vi "UHR-Fleezers Control (host) - 10.6.vi"() -> ()   [LabVIEW 2011] (continued)
                                n777 = property on="Green Laser ON/Interlacing" class="Bool (strict)"("Val(Sgnl)"=TRUE ("Green Laser ON/Interlacing")) -> ()  [unwired: 2 in, 2 out]
                                }
                                }
                                }
                                frame #2 {
                                n778 = Wait (ms)(milliseconds to wait=u32 500) -> ()  [unwired: 1 out]
                                }
                                frame #3 {
                                n779 = local write "Start Saving"("Save at end (5, 6)") -> ()
                                }
                                }
                                }
                                frame #2 {
                                n780 = local read "Bead Sep. Int. Time (s)"() -> (w1214:dbl)
                                n781 = Multiply(x=w1214, y=1000.0) -> (x*y=w1213:dbl)
                                n782 = Wait (ms)(milliseconds to wait=w1213) -> ()  [unwired: 1 out]
                                }
                                frame #3 {
                                n783 = property on="Remove Offset" class="Bool (strict)"("Val(Sgnl)"=TRUE ("Value (Signaling)")) -> ()  [unwired: 2 in, 2 out]
                                }
                                }
                                }
                                }
                                }
                                }
                                }
                                }
                                }
                                frame "2", Default {
                                }
                              }
                            }
                          }
                        }
                      }
                      "Tether" <- "Tether Alarm?"
                    }
                  }
                }
                frame #2 {
                  n784 = local read "Oscillate Set 1"() -> (w1221:bool)
                  n785 = local read "Stop All"() -> (w1219:bool)
                  n786 = Or(x=w1221, y=w1216) -> (x .or. y?=w1218:bool)
                  n787 = Not(x=w1218) -> (.not. x?=w1220:bool)
                  n788 = Compound Arithmetic op=OR(w1219, w1220) -> (w1217:bool)
                }
              }
              n789 = node-c288() -> ()  [unwired: 2 out]
            }
            n790 = node-c288(w1062) -> ()  [unwired: 1 out]
          }
        }
      }
      event "Fl. Triggered...": Value Change {
        n791 = event-data() -> ()  [unwired: 7 out]
        n792 = case shown="True" "Fl. Triggered..." {
          frame False {
          }
          frame True {
            n793 = node-c288() -> (w1231:T21)  [unwired: 4 out]
            n794 = timed-loop {
              timing: w1231 -> [_]
              timing-out: [_] -> w1230
              tunnel: "Action" -> [w1235]
              shift-right: [w1232] -> _
              shift-left: u8 255 -> [w1234]
              stop <- w1236 stop-if-true
              n795 = node-c288() -> ()  [unwired: 2 out]
              n796 = flat-sequence {
                tunnel: w1235 -> [w1248]
                tunnel: w1234 -> [w1245]
                tunnel: [w1244] -> w1233
                tunnel: [w1334] -> w1236
                tunnel: w1233 -> [w1333]
                tunnel: [w1333] -> w1232
                frame #0 {
                  n797 = local read "Delta Fl. 2"() -> (w1239:dbl)
                  n798 = local read "Delta Fl. 1"() -> (w1240:dbl)
                  n799 = Select(t=w1240, s="APD to Watch", f=w1239) -> (s? t:f=w1238:dbl)
                  n800 = Multiply(x="Fl. Delta Thresh. (kHz)", y=1000.0) -> (x*y=w1247:dbl)
                  n801 = Greater?(x=w1238, y=w1247) -> (0:w1242:bool)
                  n802 = Or(x="Force Yank", y=w1242) -> (x .or. y?=w1243:bool)
                  n803 = case shown="True" w1243 {
                    tunnel: w1248 -> [_ w1258]
                    tunnel: w1245 -> [w1250 w1254]
                    tunnel: [w1250 w1251] -> w1244
                    frame False {
                    }
                    frame True {
                      n804 = flat-sequence {
                        tunnel: w1255 -> [w1264]
                        tunnel: [w1264] -> w1259
                        tunnel: w1258 -> [w1263]
                        tunnel: [w1263] -> w1257
                        tunnel: [w1262] -> w1256
                        tunnel: w1254 -> [w1261]
                        tunnel: [w1260] -> w1253
                        tunnel: w1259 -> [w1289]
                        tunnel: w1257 -> [w1288]
                        tunnel: w1256 -> [w1287]
                        tunnel: w1253 -> [w1286]
                        tunnel: [w1286] -> w1252
                        tunnel: w1252 -> [w1331]
                        tunnel: [w1331] -> w1251
                        frame #0 {
                          n805 = call <vilib>:"Beep.vi"() -> ()  [unwired: 3 in, 9 out]
                          n806 = local write "Waiting"(FALSE ("Waiting")) -> ()
                          n807 = Increment(x=w1261) -> (x+1=w1260:u8)
                          n808 = case shown="\"Yank\"" w1263 {
                            tunnel: w1260 -> [_ _ w1270]
                            frame "Image" {
                              n809 = property on="Confocal Image" class="Bool (strict)"("Val(Sgnl)"=TRUE ("Value (Signaling)")) -> ()  [unwired: 2 in, 2 out]
                            }
                            frame "Alarm", Default {
                            }
                            frame "Yank" {
                              n810 = flat-sequence {
                                tunnel: w1270 -> [w1273]
                                tunnel: [w1272] -> w1269
                                tunnel: ["N Array El"] -> w1268
                                tunnel: w1269 -> [w1283]
                                tunnel: w1268 -> [w1279]
                                frame #0 {
                                n811 = Multiply(x="Yank Delay (s)", y=1000.0) -> (x*y=w1276:dbl)
                                n812 = Quotient & Remainder(x=w1273, y="N Array El") -> (x-y*floor(x/y)=w1272:u8)  [unwired: 1 out]
                                n813 = Wait (ms)(milliseconds to wait=w1276) -> ()  [unwired: 1 out]
                                }
                                frame #1 {
                                n814 = Random Number (0-1)() -> (number: 0 to 1=w1280:dbl)
                                n815 = Multiply(x=w1279, y=w1280) -> (x*y=w1278:dbl)
                                n816 = Round Toward -Infinity(1:w1278) -> (0:w1277:dbl)
                                n817 = Select(t=w1277, s="Random Choice", f=w1283) -> (s? t:f=w1281:dbl)
                                n818 = Index Array(array="Yank to Delta Array (MHz)", index=w1281) -> (element=w1284:dbl)
                                n819 = property on="Trap Delta (MHz)" class="DigNum (strict)"("Val(Sgnl)"=w1284) -> ()  [unwired: 2 in, 2 out]
                                }
                              }
                            }
                          }
                          n820 = local read "Time (s)"() -> (w1262:dbl)
                          "Fl. High" <- TRUE ("Yanking")
                        }
                        frame #1 {
                          n821 = node-c288() -> (w1291:T21)  [unwired: 4 out]
                          n822 = timed-loop {
                            timing: w1291 -> [_]
                            timing-out: [_] -> w1290
                            tunnel: w1289 -> [w1307]
                            tunnel: w1288 -> [w1305]
                            tunnel: w1287 -> [w1304]
                            stop <- w1306 stop-if-true
                            n823 = node-c288() -> ()  [unwired: 2 out]
                            n824 = local read "Fl. Delta Thresh. (kHz)"() -> (w1299:dbl)
                            n825 = local read "Fl. Triggered..."() -> (w1308:bool)
                            n826 = local read "Delta Fl. 1"() -> (w1295:dbl)
                            n827 = local read "Delta Fl. 2"() -> (w1293:dbl)
                            n828 = local read "Stop All"() -> (w1302:bool)
                            n829 = local read "APD to Watch"() -> (w1294:bool)
                            n830 = Select(t=w1295, s=w1294, f=w1293) -> (s? t:f=w1292:dbl)
                            n831 = Not(x=w1308) -> (.not. x?=w1303:bool)
                            n832 = Multiply(x=w1299, y=1000.0) -> (x*y=w1298:dbl)
                            n833 = Negate(x=w1298) -> (-x=w1297:dbl)
                            n834 = Less?(x=w1292, y=w1297) -> (x < y?=w1301:bool)
                            n835 = Compound Arithmetic op=OR(w1301, w1302, w1303, "Force Reset") -> (w1306:bool)
                            n836 = case shown="True" w1306 {
                              tunnel: w1307 -> [_ w1319]
                              tunnel: w1305 -> [_ w1318]
                              tunnel: w1304 -> [_ w1316]
                              frame False {
                              }
                              frame True {
                                n837 = case shown="\"Yank\"" w1318 {
                                tunnel: w1319 -> [_ w1320]
                                frame "Image", Default {
                                }
                                frame "Yank" {
                                n838 = flat-sequence {
                                tunnel: [w1325] -> w1321
                                tunnel: w1320 -> [w1325]
                                tunnel: w1321 -> [w1326]
                                frame #0 {
                                n839 = local read "Yank Delay (s)"() -> (w1324:dbl)
                                n840 = Multiply(x=w1324, y=1000.0) -> (x*y=w1322:dbl)
                                n841 = Wait (ms)(milliseconds to wait=w1322) -> ()  [unwired: 1 out]
                                }
                                frame #1 {
                                n842 = property on="Trap Delta (MHz)" class="DigNum (strict)"("Val(Sgnl)"=w1326) -> ()  [unwired: 2 in, 2 out]
                                }
                                }
                                }
                                }
                                n843 = local read "Time (s)"() -> (w1317:dbl)
                                n844 = Subtract(x=w1317, y=w1316) -> (x-y=w1313:dbl)
                                "Duration (s)" <- w1313
                                n845 = Number To Decimal String(number=w1313, width (-)=i16 0) -> (decimal integer string=w1311:string)
                                n846 = Concatenate Strings(w1311, " s fluorescence event." ("string")) -> (w1309:string)
                                n847 = local read "Messages"() -> (w1315:string)
                                n848 = call "Update messages.vi"("Message to add"=w1309, "Old message string"=w1315) -> ("New message string"=w1314:string)
                                n849 = call <vilib>:"Beep.vi"() -> ()  [unwired: 3 in, 9 out]
                                n850 = local write "Messages"(w1314) -> ()
                              }
                            }
                            n851 = node-c288() -> ()  [unwired: 2 out]
                          }
                          n852 = node-c288(w1290) -> ()  [unwired: 1 out]
                        }
                        frame #2 {
                          n853 = local write "Fl. High"(FALSE ("Yanking")) -> ()
                        }
                      }
                      n854 = local read "Trap Delta (MHz)"() -> (w1255:dbl)
                    }
                  }
                }
                frame #1 {
                  n855 = local read "Stop All"() -> (w1337:bool)
                  n856 = local read "Fl. Triggered..."() -> (w1335:bool)
                  n857 = Not(x=w1335) -> (.not. x?=w1336:bool)
                  n858 = Or(x=w1336, y=w1337) -> (x .or. y?=w1334:bool)
                  n859 = Not(x=w1334) -> (.not. x?=→"Waiting":bool)
                }
              }
              n860 = node-c288() -> ()  [unwired: 2 out]
            }
            n861 = node-c288(w1230) -> ()  [unwired: 1 out]
          }
        }
      }
      event "Stop All": Value Change {
        n862 = event-data() -> ()  [unwired: 7 out]
        n863 = local read "Stop All"() -> (w1343:bool)
      }
    }
    n864 = node-c288() -> ()  [unwired: 2 out]
  }
  n865 = timed-loop "Control parameters (event loop)" {
    tunnel: w50 -> [w1352]
    shift-right: [w1351] -> _
    shift-left: errorcluster {"status"=FALSE, "code"=0, "source"=""} ("error out") -> [w1350]
    tunnel: [w1349] -> _
    timing: w92 -> [_]
    timing-out: [_] -> w91
    tunnel: w64 -> [w1348]
    tunnel: w4 -> [w1347]
    tunnel: w3 -> [w1346]
    tunnel: w2 -> [w1345]
    tunnel: w1 -> [w1344]
    stop <- w1349 stop-if-true
    n866 = node-c288() -> ()  [unwired: 2 out]
    n867 = event shown="[56] \"Retract Pump 3\": Value Change" {
      selector: _ -> [_ _ _ _ _ _ _ _ _ _ _ _ _ _ _ _ _ _ _ _ _ _ _ _ _ _ _ _ _ _ _ _ _ _ _ _ _ _ _ _ _ _ _ _ _ _ _ _ _ _ _ _ _ _ _ _ _ _ _ _ _ _ _ _ _ _ _ _ _ _ _ _ _]
      dyn-events: _ -> [_ _ _ _ _ _ _ _ _ _ _ _ _ _ _ _ _ _ _ _ _ _ _ _ _ _ _ _ _ _ _ _ _ _ _ _ _ _ _ _ _ _ _ _ _ _ _ _ _ _ _ _ _ _ _ _ _ _ _ _ _ _ _ _ _ _ _ _ _ _ _ _ _]
      timeout: _ -> [_ _ _ _ _ _ _ _ _ _ _ _ _ _ _ _ _ _ _ _ _ _ _ _ _ _ _ _ _ _ _ _ _ _ _ _ _ _ _ _ _ _ _ _ _ _ _ _ _ _ _ _ _ _ _ _ _ _ _ _ _ _ _ _ _ _ _ _ _ _ _ _ _]
      tunnel: w1352 -> [w1390 _ _ _ w1428 _ w1450 _ _ _ _ w1516 _ _ w1559 w1565 w1570 w1576 w1612 w1630 w1637 w1648 w1652 w1663 w1674 w1685 w1696 w1707 w1718 w1745 w1839 w1846 w1884 _ w1919 w1923 w1934 w1938 w1942 _ w1950 _ _ _ _ _ _ _ _ _ _ _ _ _ _ _ _ _ w2328 _ w2345 _ w2352 w2370 _ w2377 w2385 w2400 w2411 w2414 w2419 _ w2438]
      tunnel: [w1389 _ _ _ w1418 _ w1449 _ _ w1481 _ w1495 _ _ w1558 w1561 w1567 w1573 w1611 w1628 w1636 w1646 _ w1657 w1668 w1679 w1690 w1701 w1712 w1743 w1837 w1844 w1882 _ w1917 w1921 w1924 w1936 w1940 _ w1948 _ _ _ _ _ _ _ _ _ _ _ _ _ _ _ _ _ w2326 _ _ _ _ w2367 _ _ _ _ _ _ _ _ _] -> w1351
      tunnel: w1350 -> [w1388 _ _ _ w1427 _ w1448 _ _ w1481 _ w1515 _ _ w1557 w1560 w1566 w1572 w1610 w1629 w1635 w1647 w1651 w1662 w1673 w1684 w1695 w1706 w1717 w1744 w1838 w1845 w1883 _ w1918 w1922 w1933 w1937 w1941 _ w1949 _ _ _ _ _ _ _ _ _ _ _ _ _ _ _ _ _ w2327 _ w2344 _ w2351 w2369 _ w2376 w2384 w2399 w2410 w2413 w2418 _ w2437]
      tunnel: [_ _ _ _ _ _ _ _ _ w1480 _ _ _ _ _ _ _ _ _ _ _ _ _ _ _ _ _ _ _ _ _ _ _ _ _ _ _ _ _ _ _ _ _ _ _ _ _ _ _ _ _ _ _ _ _ _ _ _ _ _ _ _ _ _ _ _ _ _ _ _ _ _ _] -> w1349
      tunnel: [_ _ _ _ _ _ _ "Round T1 X" _ _ _ _ _ _ _ _ _ _ _ _ _ _ _ _ _ _ _ _ _ _ _ _ _ _ _ _ _ _ _ _ _ _ _ _ _ _ _ _ _ _ _ _ _ _ _ _ _ _ _ _ _ _ _ _ _ _ _ _ _ _ _ _ _] -> _
      tunnel: [_ _ _ "Adjust Scale\nto Mean" _ _ _ _ _ _ _ _ _ _ _ _ _ _ _ _ _ "Test ttrig" _ _ _ _ _ _ _ _ _ _ _ _ _ _ _ _ _ _ _ _ _ _ _ _ _ _ "Flush Sample" "Flush Pump 3" "Flush Pump 1" "Clear Volume" _ _ _ _ _ _ _ _ _ _ _ _ _ _ _ _ _ _ _ _ _] -> _
      tunnel: [_ _ _ _ _ _ _ _ "Round T2 X" _ "Delayed Interlace Start" _ _ _ _ _ _ _ _ _ _ _ _ _ _ _ _ _ _ _ _ _ _ _ _ _ _ _ _ _ _ _ _ _ _ _ _ _ _ _ _ _ _ _ _ _ _ _ _ _ _ _ _ _ _ _ _ _ _ _ _ _ _] -> _
      tunnel: w1348 -> [_ _ _ _ _ _ _ _ _ _ _ _ _ _ _ _ _ _ _ _ _ _ _ _ _ _ _ _ _ _ _ _ _ _ _ _ _ _ _ _ _ _ _ _ w2107 w2114 w2121 w2126 w2135 _ _ w2241 _ _ _ _ _ _ _ _ _ _ _ _ _ _ _ _ _ _ _ _ _]
      tunnel: w1347 -> [_ _ _ _ _ _ _ _ _ _ _ _ _ _ _ _ _ _ _ _ _ _ _ _ _ _ _ _ _ _ _ _ _ _ _ _ _ _ _ _ _ _ w2024 _ _ _ _ _ _ w2179 _ _ w2247 _ w2256 _ w2270 _ _ _ _ _ _ _ _ _ _ _ _ _ _ _ _]
      tunnel: w1346 -> [_ _ _ _ _ _ _ _ _ _ _ _ _ _ _ _ _ _ _ _ _ _ _ _ _ _ _ _ _ _ _ _ _ _ _ _ _ _ _ _ _ _ _ _ _ _ _ _ _ _ _ _ _ _ _ _ _ _ _ _ _ _ _ _ _ _ _ _ _ _ _ _ _]
      tunnel: w1345 -> [_ _ _ _ _ _ _ _ _ _ _ _ _ _ _ _ _ _ _ _ _ _ _ _ _ _ _ _ _ _ _ _ _ _ _ _ _ _ _ _ _ w1961 _ _ _ _ _ _ _ _ w2209 _ _ w2252 _ w2263 _ w2295 _ _ _ _ _ _ _ _ _ _ _ _ _ _ _]
      tunnel: w1344 -> [_ _ _ _ _ _ _ _ _ _ _ _ _ _ _ _ _ _ _ _ _ _ _ _ _ _ _ _ _ _ _ _ _ _ _ _ _ _ _ _ _ _ _ _ _ _ _ _ _ _ _ _ _ _ _ _ _ _ _ _ _ _ _ _ _ _ _ _ _ _ _ _ _]
      event "AI Count (ticks)", "Sets to FIFO (Traps)", "Save ave N", "FPGA Ave.", "# Samples/channel", "N sets to save": Value Change {
        # "So that if 'Save ave N' is updated, the AOD scanning code updates too."
        n868 = event-data() -> ()  [unwired: 6 out]
        n869 = local read "AI Count (ticks)"() -> (w1370:u32)
        n870 = Boolean To (0,1)(Boolean="Sets to FIFO (Traps)") -> (0, 1=w1380:cluster{"Set 1":i16, "Set 2":i16, "Set 3":i16})
        n871 = xnode "Read/Write Control"("FPGA VI Reference In"=w1390, "error in"=w1388, "ai count"=w1370, "AI1 Sets to FIFO"="Sets to FIFO (Traps)", "N of AI1 Int Acq Sets"="N Acq Sets (Traps + Fl.)") -> ("error out"=w1389:errorcluster)  [unwired: 1 out]
        n872 = Cluster To Array(cluster=w1380) -> (array=w1379:i16[])
        n873 = To Unsigned Long Integer(number=w1379) -> (unsigned 32bit integer=w1359:u32[])
        n874 = local read "Scan steps (AOD)"() -> (w1381:u64)
        n875 = Multiply(x=w1370, y="N Acq Sets (Traps + Fl.)") -> (x*y=w1368:u32)
        n876 = Divide(x=40000000.0, y=w1370) -> (x/y=w1362:dbl)
        "AI rate (Hz)" <- w1362
        "Ave. Rate (Hz)" <- w1362
        n877 = Add Array Elements(numeric array=w1359) -> (sum=w1371:u32)
        "Trap Sets" <- w1371
        n878 = Reciprocal(x=w1362) -> (1/x=→"Ave. Period (s)":dbl)
        n879 = property on="Scan steps (AOD)" class="DigNum (strict)"("Val(Sgnl)"=w1381) -> ()  [unwired: 2 in, 2 out]
        n880 = Divide(x=w1362, y="N Acq Sets (Traps + Fl.)") -> (x/y=w1385:dbl)
        "Data Rate (Hz)" <- w1385
        n881 = Reciprocal(x=w1385) -> (1/x=→"Data Period (s)":dbl)
        n882 = local read "Save ave N"() -> (w1384:dbl)
        n883 = Divide(x=w1385, y=w1384) -> (x/y=w1383:dbl)
        "Save Data Rate (Hz)" <- w1383
        n884 = Reciprocal(x=w1383) -> (1/x=→"Save Data Period (s)":dbl)
        n885 = Multiply(x=w1368, y="# Samples/trap") -> (x*y=w1366:u32)
        "Counts/DMA" <- w1366
        n886 = property on="Trap Disp. Downsample" class="DigNum (strict)"("Maximum"="# Samples/trap") -> ()  [unwired: 2 in, 2 out]
        n887 = Multiply(x=w1371, y="# Samples/trap") -> (x*y=w1360:u32)
        "# Samples/channel" <- w1360
        n888 = Multiply(x=w1360, y=u32 8) -> (x*y=→"Trap AI Elements/DMA read":u32)
        n889 = local read "APD Int. Count"() -> (w1367:u32)
        n890 = Multiply(x=w1360, y=u32 3) -> (x*y=→"Trap Pos Elements/DMA read":u32)
        n891 = Divide(x=w1366, y=w1367) -> (x/y=w1357:dbl)
        "APD Samples/FIFO Acq." <- w1357
        n892 = Divide(x=w1366, y=40000000.0) -> (x/y=w1364:dbl)
        "DMA Update Period (s)" <- w1364
        n893 = Multiply(x=2.0, y=w1357) -> (x*y=→"APD Elements/DMA read":dbl)
        n894 = property on="APD Disp. Downsample" class="DigNum (strict)"("Maximum"=w1357) -> ()  [unwired: 2 in, 2 out]
        n895 = local read "N sets to save"() -> (w1377:u32)
        n896 = Multiply(x=w1364, y=w1377) -> (x*y=→"Total Time (s)":dbl)
        "FPGA Averaging" <- FALSE ("FPGA Averaging")
      }
      event "Remove Offset": Value Change {
        n897 = event-data() -> ()  [unwired: 7 out]
        n898 = local write "Remove Offset"(FALSE ("Remove Offset")) -> ()
        n899 = local read "Bead Mean (nm)"() -> (w1392:dbl)
        n900 = local read "Offset (nm)"() -> (w1393:dbl)
        n901 = Add(x=w1392, y=w1393) -> (x+y=w1391:dbl)
        n902 = local write "Offset (nm)"(w1391) -> ()
        n903 = disable-structure shown="Disabled" {
          frame Disabled {
            n904 = local read "Bead Mean (nm)"() -> (w1398:dbl)
            n905 = Add(y=w1398) -> (x=w1397:dbl, x+y=w1396:dbl)
            n906 = Subtract(x=w1398, y=w1397) -> (x-y=w1395:dbl)
            n907 = property on="Bead Separation" class="WFChart (strict)"("YScale.Minimum"=w1395) -> ()  [unwired: 2 in, 2 out]
            n908 = property on="Bead Separation" class="WFChart (strict)"("YScale.Maximum"=w1396) -> ()  [unwired: 2 in, 2 out]
          }
          frame Enabled {
          }
        }
      }
      event "Detector Type": Value Change {
        n909 = event-data() -> ()  [unwired: 7 out]
        n910 = local read "AI labels"() -> (w1399:string[])
        n911 = property on="High Res. Display" class="Ring (strict)"("Strings []"=w1399) -> ()  [unwired: 2 in, 2 out]
        n912 = Build Array (concatenate)(w1399, "none") -> (w1400:string[])
        n913 = property on="FFT 1 Choice 1" class="Ring (strict)"("Strings []"=w1400) -> ()  [unwired: 2 in, 2 out]
        n914 = property on="FFT 1 Choice 2" class="Ring (strict)"("Strings []"=w1400) -> ()  [unwired: 2 in, 2 out]
        n915 = property on="FFT 2 Choice 1" class="Ring (strict)"("Strings []"=w1400) -> ()  [unwired: 2 in, 2 out]
        n916 = property on="FFT 2 Choice 2" class="Ring (strict)"("Strings []"=w1400) -> ()  [unwired: 2 in, 2 out]
        n917 = Bundle("APD 1", "APD 2") -> (w1403:cluster{string, string})  [unwired: 1 out]
        n918 = Cluster To Array(cluster=w1403) -> (array=w1401:string[])
        n919 = Build Array (concatenate)(w1401, w1400) -> (w1405:string[])
        n920 = Array Size(array=w1405) -> (size(s)=w1406:i32)
        n921 = property on="Signals to Plot" class="LstBox (strict)"("Item Names"=w1405) -> ()  [unwired: 2 in, 2 out]
        n922 = property on="Signals to Plot" class="LstBox (strict)"("Number of Rows"=w1406) -> ()  [unwired: 2 in, 2 out]
        n923 = property on="All Signals" class="WFChart (strict)"("LegNumRows"=w1406) -> ()  [unwired: 2 in, 2 out]
      }
      event "Adjust Scale\nto Mean": Value Change {
        n924 = event-data() -> ()  [unwired: 7 out]
        n925 = local read "APD 1 Rate (Hz)"() -> (w1415:dbl)
        n926 = Multiply(x=1000.0, y="Above (kHz)") -> (x*y=w1413:dbl)
        n927 = Multiply(x=1000.0, y="Below (kHz)") -> (x*y=w1411:dbl)
        n928 = Add(x=w1413, y=w1415) -> (x+y=w1408:dbl)
        n929 = Subtract(x=w1415, y=w1411) -> (x-y=w1409:dbl)
        n930 = property on="APD Chart" class="WFChart (strict)"("YScale.Minimum"=w1409) -> ()  [unwired: 2 in, 2 out]
        n931 = property on="APD Chart" class="WFChart (strict)"("YScale.Maximum"=w1408) -> ()  [unwired: 2 in, 2 out]
      }
      event "Phase adj. (AI1)", "+ phase (AI1)", "- phase (AI1)": Value Change {
        n932 = event-data() -> ()  [unwired: 7 out]
        n933 = Negate(x="Phase adj. (AI1)") -> (-x=w1425:i16)
        n934 = Select(t=w1425, s="- phase (AI1)", f="Phase adj. (AI1)") -> (s? t:f=w1424:i16)
        n935 = xnode "Read/Write Control"("FPGA VI Reference In"=w1428, "error in"=w1427, "Phase count adjustment"=w1424) -> ("FPGA VI Reference Out"=w1423:T19, "error out"=w1422:errorcluster)
        n936 = Or(x="- phase (AI1)", y="+ phase (AI1)") -> (x .or. y?=w1419:bool)
        n937 = xnode "Read/Write Control"("FPGA VI Reference In"=w1423, "error in"=w1422, "+ phase"=w1419) -> ("error out"=w1418:errorcluster)  [unwired: 1 out]
      }
      event "Signals to Plot": Double Click {
        w1431 = u32 9868950 ("Color Box")
        n938 = event-data() -> ("Row"=w1433:i32)  [unwired: 9 out]
        n939 = property on="All Signals" class="WFChart (strict)"("Active Plot"=w1433) -> (error out=w1444:errorcluster)  [unwired: 2 in, 1 out]
        n940 = property on="All Signals" class="WFChart (strict)" props=["Plot", "Visible?", "Plot", "Plot Color"](error in=w1444) -> (error out=w1443:errorcluster, "Plot.Visible?"=w1442:bool)  [unwired: 1 in, 2 out]
        n941 = Select(t=FALSE ("Plot.Visible"), s=w1442, f=TRUE ("Plot.Visible")) -> (s? t:f=w1437:bool)
        n942 = property on="All Signals" class="WFChart (strict)"(error in=w1443, "Plot.Visible?"=w1437) -> (error out=w1439:errorcluster)  [unwired: 1 in, 1 out]
        n943 = property on="All Signals" class="WFChart (strict)"(error in=w1439) -> (error out=w1434:errorcluster, "Plot.Plot Color"=w1438:u32)  [unwired: 1 in, 1 out]
        n944 = property on="Signals to Plot" class="LstBox (strict)"(error in=w1434, "Active Row"=w1433) -> (error out=w1432:errorcluster)  [unwired: 1 in, 1 out]
        n945 = Select(t=w1438, s=w1437, f=u32 0) -> (s? t:f=w1435:u32)
        n946 = property on="Signals to Plot" class="LstBox (strict)"(error in=w1432, "CellFontColor"=w1435, "SelColor"=w1431, "CellBG"=w1431, "CellFontSize"=u32 20 ("Active Row:Cell Font:Size"), "CellFontBold"=TRUE ("Active Row:Cell Font:Bold")) -> ()  [unwired: 1 in, 2 out]
      }
      event "BD 1 Frequency 1 (MHz)", "BD 1 Frequency 2 (MHz)", "BD 1 Frequency 3 (MHz)", "BD 2 Frequency 1 (MHz)", "BD 2 Frequency 2 (MHz)", "BD 2 Frequency 3 (MHz)", "Trap Delta (MHz)": Value Change {
        n947 = event-data() -> ("CtlRef"=w1447:refnum<vi>)  [unwired: 6 out]
        n948 = control-ref of="Trap Delta (MHz)"() -> (w1446:refnum<vi>)
        n949 = Equal?(x=w1446, y=w1447) -> (x = y?=w1445:bool)
        n950 = case shown="False" "Oscillate Set 1" {
          tunnel: w1450 -> [w1470 _]
          tunnel: [w1469 w1473] -> w1449
          tunnel: w1448 -> [w1468 w1473]
          tunnel: w1445 -> [w1453 _]
          frame False {
            n951 = local read "BD 1 Frequency 2 (MHz)"() -> (w1457:dbl)
            n952 = local read "BD 1 Frequency 1 (MHz)"() -> (w1455:dbl)
            n953 = Subtract(x=w1457, y="Trap Delta (MHz)") -> (x-y=w1454:dbl)
            n954 = Select(t=w1454, s=w1453, f=w1455) -> (s? t:f=w1452:dbl)
            n955 = local read "Y RF Frequency Limits (MHz)"() -> (w1458:T16)
            n956 = local read "X RF Frequency Limits (MHz)"() -> (w1459:T16)
            n957 = local read "BD 1 Frequency 3 (MHz)"() -> (w1471:dbl)
            n958 = local write "BD 1 Frequency 1 (MHz)"(w1452) -> ()
            n959 = local read "BD 2 Frequency 1 (MHz)"() -> (w1462:dbl)
            n960 = local read "BD 2 Frequency 2 (MHz)"() -> (w1461:dbl)
            n961 = local read "BD 2 Frequency 3 (MHz)"() -> (w1472:dbl)
            n962 = call "set RF board frequency - interlace.vi"("Board 2 Frequency Limits"=w1458, "Board 1 Frequency Limits"=w1459, "error in"=w1468, "FPGA VI Reference In"=w1470, "Board 2 Frequency 3 (MHz)"=w1472, "Board 1 Frequency 3 (MHz)"=w1471, "Board 2 Frequency 2 (MHz)"=w1461, "Board 2 Frequency 1 (MHz)"=w1462, "Board 1 Frequency 2 (MHz)"=w1457, "Board 1 Frequency 1  (MHz)"=w1452) -> ("error out"=w1469:errorcluster)  [unwired: 1 out]
            n963 = Subtract(x=w1462, y=w1461) -> (x-y=w1466:dbl)
            n964 = Subtract(x=w1452, y=w1457) -> (x-y=w1467:dbl)
            n965 = Square(x=w1466) -> (x^2=w1464:dbl)
            n966 = Square(x=w1467) -> (x^2=w1465:dbl)
            n967 = Add(x=w1465, y=w1464) -> (x+y=w1463:dbl)
            n968 = Square Root(x=w1463) -> (sqrt(x)=w1460:dbl)
            n969 = local write "Trap Delta (MHz)"(w1460) -> ()
            n970 = property on="Initial delta (MHz)" class="DigNum (strict)"("Val(Sgnl)"=w1460) -> ()  [unwired: 2 in, 2 out]
          }
          frame True {
          }
        }
      }
      event "Round T1 X": Value Change {
        n971 = event-data() -> ()  [unwired: 7 out]
        n972 = local read "BD 1 Frequency 1 (MHz)"() -> (w1476:dbl)
        n973 = Round To Nearest(number=w1476) -> (nearest integer value=w1475:dbl)
        n974 = property on="BD 1 Frequency 1 (MHz)" class="DigNum (strict)"("Val(Sgnl)"=w1475) -> ()  [unwired: 2 in, 2 out]
      }
      event "Round T2 X": Value Change {
        n975 = event-data() -> ()  [unwired: 7 out]
        n976 = local read "BD 1 Frequency 2 (MHz)"() -> (w1478:dbl)
        n977 = Round To Nearest(number=w1478) -> (nearest integer value=w1477:dbl)
        n978 = property on="BD 1 Frequency 2 (MHz)" class="DigNum (strict)"("Val(Sgnl)"=w1477) -> ()  [unwired: 2 in, 2 out]
      }
      event "Stop All": Value Change {
        n979 = event-data() -> ()  [unwired: 7 out]
        n980 = local read "Stop All"() -> (w1480:bool)
      }
      event "Delayed Interlace Start": Value Change {
        n981 = event-data() -> ()  [unwired: 7 out]
        n982 = flat-sequence {
          frame #0 {
            n983 = Multiply(x="Delay to Interlace (s)", y=1000.0) -> (x*y=w1483:dbl)
            n984 = Wait (ms)(milliseconds to wait=w1483) -> ()  [unwired: 1 out]
          }
          frame #1 {
            n985 = property on="Green laser mode" class="RadioBtnsControl (strict)"("Val(Sgnl)"=enum32{"Laser ON", "Laser OFF", "Interlace"}."Interlace" ("Value (Signaling)")) -> ()  [unwired: 2 in, 2 out]
          }
        }
      }
      event "BD 1 Amplitude 1 (%)", "BD 1 Amplitude 2 (%)", "BD 1 Amplitude 3 (%)", "BD 2 Amplitude 1 (%)", "BD 2 Amplitude 2 (%)", "BD 2 Amplitude 3 (%)", "Trap 1 ON", "Trap 2 ON", "Trap 3 ON", "Feedback On/Off", "All FB On/Off": Value Change {
        w1507 = i16 1 ("f")
        n986 = event-data() -> ()  [unwired: 7 out]
        n987 = local write "Trap 1 (ON/OFF)"("Trap 1 ON") -> ()
        n988 = local write "Trap 2 (ON/OFF)"("Trap 2 ON") -> ()
        n989 = Boolean To (0,1)(Boolean="Trap 3 ON") -> (0, 1=w1508:i16)
        n990 = Boolean To (0,1)(Boolean="Trap 1 ON") -> (0, 1=w1509:i16)
        n991 = Boolean To (0,1)(Boolean="Trap 2 ON") -> (0, 1=w1510:i16)
        n992 = Select(t=w1510, s="Trap ON/OFF X or Y Amp?", f=w1507) -> (s? t:f=w1505:i16)
        n993 = Select(t=w1509, s="Trap ON/OFF X or Y Amp?", f=w1507) -> (s? t:f=w1506:i16)
        n994 = Select(t=w1508, s="Trap ON/OFF X or Y Amp?", f=w1507) -> (s? t:f=w1504:i16)
        n995 = Select(t=w1507, s="Trap ON/OFF X or Y Amp?", f=w1510) -> (s? t:f=w1502:i16)
        n996 = Select(t=w1507, s="Trap ON/OFF X or Y Amp?", f=w1509) -> (s? t:f=w1503:i16)
        n997 = Select(t=w1507, s="Trap ON/OFF X or Y Amp?", f=w1508) -> (s? t:f=w1501:i16)
        n998 = And(x="All FB On/Off", y="Feedback On/Off") -> (x .and. y?=w1499:cluster{"Set 1":bool, "Set 2":bool})
        n999 = local read "BD 1 Amplitude 1 (%)"() -> (w1519:dbl)
        n1000 = local read "BD 1 Amplitude 2 (%)"() -> (w1518:dbl)
        n1001 = local read "BD 1 Amplitude 3 (%)"() -> (w1517:dbl)
        n1002 = Unbundle By Name(w1499) -> ("Set 1"=w1494:bool, "Set 2"=w1491:bool)
        n1003 = local read "Y RF Amplitude Limits (%)"() -> (w1487:T16)
        n1004 = local read "X RF Amplitude Limits (%)"() -> (w1488:T16)
        n1005 = local read "BD 2 Amplitude 1 (%)"() -> (w1520:dbl)
        n1006 = local read "BD 2 Amplitude 2 (%)"() -> (w1521:dbl)
        n1007 = local read "BD 2 Amplitude 3 (%)"() -> (w1522:dbl)
        n1008 = And(x="Trap 2 ON", y=w1491) -> (x .and. y?=w1489:bool)
        n1009 = And(x="Trap 1 ON", y=w1494) -> (x .and. y?=w1492:bool)
        n1010 = Multiply(x=w1506, y=w1519) -> (x*y=w1514:dbl)
        n1011 = Multiply(x=w1518, y=w1505) -> (x*y=w1512:dbl)
        n1012 = Multiply(x=w1517, y=w1504) -> (x*y=w1513:dbl)
        n1013 = Multiply(x=w1520, y=w1503) -> (x*y=w1523:dbl)
        n1014 = Multiply(x=w1521, y=w1502) -> (x*y=w1524:dbl)
        n1015 = Multiply(x=w1522, y=w1501) -> (x*y=w1525:dbl)
        n1016 = call "set RF board amplitude - interlace.vi"("Board 2 Amplitude Limits"=w1487, "Board 1 Amplitude Limits"=w1488, "error in"=w1515, "FPGA VI Reference In"=w1516, "Board 2 Amplitude 3 (%)"=w1525, "Board 1 Amplitude 3 (%)"=w1513, "Board 2 Amplitude 2 (%)"=w1524, "Board 2 Amplitude 1 (%)"=w1523, "Board 1 Amplitude 2 (%)"=w1512, "Board 1 Amplitude 1 (%)"=w1514) -> ("error out"=w1496:errorcluster, "FPGA VI Reference Out"=w1497:T19)
        n1017 = xnode "Read/Write Control"("FPGA VI Reference In"=w1497, "error in"=w1496, "FB On/Off Set 1"=w1492, "FB On/Off Set 2"=w1489) -> ("error out"=w1495:errorcluster)  [unwired: 1 out]
      }
      event "Load parameters": Value Change {
        n1018 = event-data() -> ()  [unwired: 7 out]
        n1019 = property on="Saved AOD Raster Scan Parameter Sets" class="Arr (strict)"() -> ("Index Values"=w1536:u32[])  [unwired: 2 in, 2 out]
        n1020 = Index Array(array=w1536, index=0) -> (element=w1533:u32)
        n1021 = local write "Load parameters"(FALSE ("Load parameters")) -> ()
        n1022 = Index Array(array="Saved AOD Raster Scan Parameter Sets", index=w1533) -> (element=w1532:T26)
        n1023 = Unbundle By Name(w1532) -> ("Scan Range AOD (nm) 2"=w1531:dbl, "Step Size AOD (nm) 2"=w1530:dbl, "Scan Speed AOD (nm/s) 2"=w1529:dbl, "Number of scans (AOD) 2"=w1528:u16)
        n1024 = flat-sequence {
          tunnel: w1531 -> [w1539]
          tunnel: w1530 -> [w1538]
          tunnel: w1529 -> [w1537]
          tunnel: w1528 -> [w1540]
          frame #0 {
            n1025 = local write "Scan Speed (nm/s)"(w1537) -> ()
            n1026 = local write "Scan Range (nm)"(w1539) -> ()
            n1027 = local write "Step Size (nm)"(w1538) -> ()
          }
          frame #1 {
            n1028 = property on="Number of F/B Scans (AOD)" class="DigNum (strict)"("Val(Sgnl)"=w1540) -> ()  [unwired: 2 in, 2 out]
          }
        }
      }
      event "Trap 1 (ON/OFF)", "Trap 2 (ON/OFF)": Value Change {
        n1029 = event-data() -> ()  [unwired: 7 out]
        n1030 = property on="Trap 2 ON" class="Bool (strict)"("Val(Sgnl)"="Trap 2 (ON/OFF)") -> ()  [unwired: 2 in, 2 out]
        n1031 = property on="Trap 1 ON" class="Bool (strict)"("Val(Sgnl)"="Trap 1 (ON/OFF)") -> ()  [unwired: 2 in, 2 out]
      }
      event "DIO count 1 (ticks)", "DIO count 2 (ticks)", "DIO count 3 (ticks)", "Interlace", "Number Interlace Sets", "Not-Interlacing Set": Value Change {
        n1032 = event-data() -> ()  [unwired: 7 out]
        n1033 = local read "DIO count 3 (ticks)"() -> (w1553:u32)
        n1034 = local read "DIO count 1 (ticks)"() -> (w1555:u32)
        n1035 = local read "DIO count 2 (ticks)"() -> (w1554:u32)
        n1036 = To Unsigned Byte Integer(number="Not-Interlacing Set") -> (unsigned 8bit integer=w1544:u8)
        n1037 = Add(x=w1544, y=u8 1) -> (x+y=w1548:u8)
        n1038 = xnode "Read/Write Control"("FPGA VI Reference In"=w1559, "error in"=w1557, "DIO count 1 (ticks)"=w1555, "DIO count 2 (ticks)"=w1554, "DIO count 3 (ticks)"=w1553, "Interlace ON/OFF"="Interlace", "Number Interlace Cycles"="Number Interlace Sets", "Interlace Off Parameters"=w1548) -> ("error out"=w1558:errorcluster)  [unwired: 1 out]
        n1039 = Build Array(w1555, w1554, w1553) -> (w1546:u32[])
        n1040 = Split 1D Array(array=w1546, index="Number Interlace Sets") -> (first subarray=w1556:u32[])  [unwired: 1 out]
        n1041 = Index Array(array=w1546, index=w1544) -> (element=w1545:u32)
        n1042 = Add Array Elements(numeric array=w1556) -> (sum=w1550:u32)
        n1043 = Select(t=w1550, s="Interlace", f=w1545) -> (s? t:f=→"Total Counts (ticks)":u32)
      }
      event "Reset Feedback": Value Change {
        n1044 = event-data() -> ()  [unwired: 7 out]
        n1045 = Unbundle By Name("Reset Feedback") -> ("Set 1"=w1563:bool, "Set 2"=w1562:bool)
        n1046 = xnode "Read/Write Control"("FPGA VI Reference In"=w1565, "error in"=w1560, "FB Reset Set 1"=w1563, "FB Reset Set 2"=w1562) -> ("error out"=w1561:errorcluster)  [unwired: 1 out]
      }
      event "PID Gains": Value Change {
        n1047 = event-data() -> ()  [unwired: 7 out]
        n1048 = Unbundle By Name("PID Gains") -> ("Set 1"=w1569:T14, "Set 2"=w1568:T14)
        n1049 = xnode "Read/Write Control"("FPGA VI Reference In"=w1570, "error in"=w1566, "FB Gains Set 1"=w1569, "FB Gains Set 2"=w1568) -> ("error out"=w1567:errorcluster)  [unwired: 1 out]
      }
      event "AI2 to Setpoint", "Setpoints (V)": Value Change {
        n1050 = event-data() -> ()  [unwired: 7 out]
        n1051 = xnode "Read/Write Control"("FPGA VI Reference In"=w1576, "error in"=w1572) -> ("FPGA VI Reference Out"=w1575:T19, "error out"=w1574:errorcluster, "AI2 Y Sum Set 1"=w1583:i16, "AI2 Y Sum Set 2"=w1582:i16)
        n1052 = Cluster To Array(cluster="AI2 to Setpoint") -> (array=w1586:bool[])
        n1053 = local read "AI2 (V)"() -> (w1584:cluster{"Set 1":dbl, "Set 2":dbl})
        n1054 = Or Array Elements(Boolean array=w1586) -> (logical OR=w1587:bool)
        n1055 = Bundle By Name(cluster=w1584, "Set 1"=w1583, "Set 2"=w1582) -> (w1581:cluster{"Set 1":dbl, "Set 2":dbl})
        n1056 = Divide(x=w1581, y=3276.7) -> (x/y=w1580:cluster{"Set 1":dbl, "Set 2":dbl})
        "AI2 (V)" <- w1580
        n1057 = case shown="True" w1587 {
          tunnel: [w1590 w1607] -> w1579
          tunnel: "AI2 to Setpoint" -> [_ w1603]
          tunnel: "Setpoints (V)" -> [w1591 w1606]
          tunnel: w1580 -> [_ w1600]
          frame False {
            n1058 = Multiply(x=3276.7, y=w1591) -> (x*y=w1592:cluster{"Set 1":dbl, "Set 2":dbl})
            n1059 = To Word Integer(number=w1592) -> (16bit integer=w1590:cluster{"Set 1":i16, "Set 2":i16})
          }
          frame True {
            n1060 = Unbundle By Name(w1600) -> ("Set 1"=w1599:dbl, "Set 2"=w1598:dbl)
            n1061 = Unbundle By Name(w1606) -> ("Set 1"=w1605:dbl, "Set 2"=w1604:dbl)
            n1062 = Unbundle By Name(w1603) -> ("Set 1"=w1602:bool, "Set 2"=w1601:bool)
            n1063 = Select(t=w1599, s=w1602, f=w1605) -> (s? t:f=w1597:dbl)
            n1064 = Select(t=w1598, s=w1601, f=w1604) -> (s? t:f=w1596:dbl)
            n1065 = Bundle By Name(cluster=w1606, "Set 1"=w1597, "Set 2"=w1596) -> (w1594:cluster{"Set 1":dbl, "Set 2":dbl})
            n1066 = local write "Setpoints (V)"(w1594) -> ()
            n1067 = Multiply(x=3276.7, y=w1594) -> (x*y=w1595:cluster{"Set 1":dbl, "Set 2":dbl})
            n1068 = To Word Integer(number=w1595) -> (16bit integer=w1607:cluster{"Set 1":i16, "Set 2":i16})
          }
        }
        n1069 = Unbundle By Name(w1579) -> ("Set 1"=w1578:i16, "Set 2"=w1577:i16)
        n1070 = xnode "Read/Write Control"("FPGA VI Reference In"=w1575, "error in"=w1574, "FB Setpoint Set 1"=w1578, "FB Setpoint Set 2"=w1577) -> ("error out"=w1573:errorcluster)  [unwired: 1 out]
      }
      event "Invert GI": Value Change {
        n1071 = event-data() -> ()  [unwired: 7 out]
        n1072 = xnode "Read/Write Control"("FPGA VI Reference In"=w1612, "error in"=w1610, "Invert GI"="Invert GI", "Invert GI 2"="Invert GI") -> ("error out"=w1611:errorcluster)  [unwired: 1 out]
      }
      event "Green FB Setpoint (mV)", "Green FB Gains", "Green FB On/Off", "Current When FB OFF (%)", "Green int current ON count adj": Value Change {
        n1073 = event-data() -> ()  [unwired: 7 out]
        n1074 = local read "Green FB Setpoint (mV)"() -> (w1619:dbl)
        n1075 = local read "Current When FB OFF (%)"() -> (w1622:dbl)
        n1076 = Multiply(x=w1619, y=3.2767) -> (x*y=w1618:dbl)
        n1077 = Multiply(x=w1622, y=655.35) -> (x*y=w1623:dbl)
        n1078 = To Unsigned Word Integer(number=w1623) -> (unsigned 16bit integer=w1621:u16)
        n1079 = local read "Green int current ON count adj"() -> (w1626:u32)
        n1080 = local read "Green FB Gains"() -> (w1625:T14)
        n1081 = local read "Green Laser ON/Interlacing"() -> (w1616:bool)
        n1082 = local read "Green laser mode"() -> (w1615:enum32{"Laser ON", "Laser OFF", "Interlace"})
        n1083 = local read "Green FB On/Off"() -> (w1627:bool)
        n1084 = Equal?(x=w1615, y=enum32{"Laser ON", "Laser OFF", "Interlace"}."Interlace") -> (x = y?=w1613:bool)
        n1085 = Compound Arithmetic op=AND(w1613, w1627, w1616) -> (w1617:bool)
        n1086 = xnode "Read/Write Control"("FPGA VI Reference In"=w1630, "error in"=w1629, "Green FB Setpoint"=w1618, "Green FB On/Off"=w1617, "Current Out"=w1621, "Green int current ON count adj"=w1626, "Green FB Gains"=w1625) -> ("error out"=w1628:errorcluster)  [unwired: 1 out]
      }
      event "Green laser mode", "Green Laser ON/Interlacing": Value Change {
        n1087 = event-data() -> ()  [unwired: 7 out]
        n1088 = case shown="True" "Green Laser ON/Interlacing" {
          tunnel: "Green laser mode" -> [_ w1644]
          tunnel: [enum32{"Laser ON", "Laser OFF", "Interlace"}."Laser OFF" ("Green laser mode") w1644] -> w1632
          tunnel: [FALSE w1640] -> w1631
          frame False {
          }
          frame True {
            n1089 = local read "Green FB On/Off"() -> (w1641:bool)
            n1090 = Equal?(x=w1644, y=enum32{"Laser ON", "Laser OFF", "Interlace"}."Interlace") -> (x = y?=w1642:bool)
            n1091 = And(x=w1642, y=w1641) -> (x .and. y?=w1640:bool)
          }
        }
        n1092 = xnode "Read/Write Control"("FPGA VI Reference In"=w1637, "error in"=w1635, "Operating Mode"=w1632, "Operating Mode 2"=w1632, "Green FB On/Off"=w1631) -> ("error out"=w1636:errorcluster)  [unwired: 1 out]
      }
      event "Test ttrig": Value Change {
        n1093 = event-data() -> ()  [unwired: 7 out]
        n1094 = xnode "Read/Write Control"("FPGA VI Reference In"=w1648, "error in"=w1647, "TTrig?"=TRUE) -> ("error out"=w1646:errorcluster)  [unwired: 1 out]
      }
      event "Neg. TTrig FPGA": Value Change {
        n1095 = event-data() -> ()  [unwired: 7 out]
        n1096 = xnode "Read/Write Control"("FPGA VI Reference In"=w1652, "error in"=w1651, "TTrig Negate Pos"="Neg. TTrig FPGA") -> ()  [unwired: 2 out]
      }
      event "- phase (APD 1 Gate)", "+ phase (APD 1 Gate)": Value Change {
        n1097 = event-data() -> ()  [unwired: 7 out]
        n1098 = local read "Phase Adj. (APD 1 Gate)"() -> (w1653:i16)
        n1099 = Negate(x=w1653) -> (-x=w1661:i16)
        n1100 = Select(t=w1661, s="- phase (APD 1 Gate)", f=w1653) -> (s? t:f=w1660:i16)
        n1101 = Or(x="- phase (APD 1 Gate)", y="+ phase (APD 1 Gate)") -> (x .or. y?=w1656:bool)
        n1102 = xnode "Read/Write Control"("FPGA VI Reference In"=w1663, "error in"=w1662, "Phase count adjustment (APD 1 Gate)"=w1660) -> ("FPGA VI Reference Out"=w1658:T19, "error out"=w1659:errorcluster)
        n1103 = xnode "Read/Write Control"("FPGA VI Reference In"=w1658, "error in"=w1659, "+ phase (APD 1 Gate)"=w1656) -> ("error out"=w1657:errorcluster)  [unwired: 1 out]
      }
      event "+ phase (APD 2 Gate)", "- phase (APD 2 Gate)": Value Change {
        n1104 = event-data() -> ()  [unwired: 7 out]
        n1105 = local read "Phase Adj. (APD 2 Gate)"() -> (w1664:i16)
        n1106 = Negate(x=w1664) -> (-x=w1672:i16)
        n1107 = Select(t=w1672, s="- phase (APD 2 Gate)", f=w1664) -> (s? t:f=w1671:i16)
        n1108 = Or(x="- phase (APD 2 Gate)", y="+ phase (APD 2 Gate)") -> (x .or. y?=w1667:bool)
        n1109 = xnode "Read/Write Control"("FPGA VI Reference In"=w1674, "error in"=w1673, "Phase count adjustment (APD 2 Gate)"=w1671) -> ("FPGA VI Reference Out"=w1669:T19, "error out"=w1670:errorcluster)
        n1110 = xnode "Read/Write Control"("FPGA VI Reference In"=w1669, "error in"=w1670, "+ phase (APD 2 Gate)"=w1667) -> ("error out"=w1668:errorcluster)  [unwired: 1 out]
      }
      event "Phase Adj. (APD Acq)", "+ phase (APD Acq)", "- phase (APD Acq)": Value Change {
        n1111 = event-data() -> ()  [unwired: 7 out]
        n1112 = local read "Phase Adj. (APD Acq)"() -> (w1677:i16)
        n1113 = Negate(x=w1677) -> (-x=w1683:i16)
        n1114 = Select(t=w1683, s="+ phase (APD Acq)", f=w1677) -> (s? t:f=w1682:i16)
        n1115 = Or(x="+ phase (APD Acq)", y="- phase (APD Acq)") -> (x .or. y?=w1678:bool)
        n1116 = xnode "Read/Write Control"("FPGA VI Reference In"=w1685, "error in"=w1684, "Phase Count Adjustment (APD Acq)"=w1682) -> ("FPGA VI Reference Out"=w1680:T19, "error out"=w1681:errorcluster)
        n1117 = xnode "Read/Write Control"("FPGA VI Reference In"=w1680, "error in"=w1681, "+ phase (APD Acq)"=w1678) -> ("error out"=w1679:errorcluster)  [unwired: 1 out]
      }
      event "Phase adj. (GI)", "+ phase (GI)", "- phase (GI)": Value Change {
        n1118 = event-data() -> ()  [unwired: 7 out]
        n1119 = Negate(x="Phase adj. (GI)") -> (-x=w1694:i16)
        n1120 = Select(t=w1694, s="+ phase (GI)", f="Phase adj. (GI)") -> (s? t:f=w1693:i16)
        n1121 = Or(x="+ phase (GI)", y="- phase (GI)") -> (x .or. y?=w1689:bool)
        n1122 = xnode "Read/Write Control"("FPGA VI Reference In"=w1696, "error in"=w1695, "Phase count adjustment (GI)"=w1693) -> ("FPGA VI Reference Out"=w1691:T19, "error out"=w1692:errorcluster)
        n1123 = xnode "Read/Write Control"("FPGA VI Reference In"=w1691, "error in"=w1692, "+ phase (GI)"=w1689) -> ("error out"=w1690:errorcluster)  [unwired: 1 out]
      }
      event "Phase adj. (GI) 2", "+ phase (GI) 2", "- phase (GI) 2": Value Change {
        n1124 = event-data() -> ()  [unwired: 7 out]
        n1125 = Negate(x="Phase adj. (GI) 2") -> (-x=w1705:i16)
        n1126 = Select(t=w1705, s="+ phase (GI) 2", f="Phase adj. (GI) 2") -> (s? t:f=w1704:i16)
        n1127 = Or(x="+ phase (GI) 2", y="- phase (GI) 2") -> (x .or. y?=w1700:bool)
        n1128 = xnode "Read/Write Control"("FPGA VI Reference In"=w1707, "error in"=w1706, "Phase count adjustment (GI) 2"=w1704) -> ("FPGA VI Reference Out"=w1702:T19, "error out"=w1703:errorcluster)
        n1129 = xnode "Read/Write Control"("FPGA VI Reference In"=w1702, "error in"=w1703, "+ phase (GI) 2"=w1700) -> ("error out"=w1701:errorcluster)  [unwired: 1 out]
      }
      event "Phase adj. (Green FB)", "- phase (Green FB)", "+ phase (Green FB)": Value Change {
        n1130 = event-data() -> ()  [unwired: 7 out]
        n1131 = Negate(x="Phase adj. (Green FB)") -> (-x=w1716:i16)
        n1132 = Select(t=w1716, s="+ phase (Green FB)", f="Phase adj. (Green FB)") -> (s? t:f=w1715:i16)
        n1133 = Or(x="+ phase (Green FB)", y="- phase (Green FB)") -> (x .or. y?=w1711:bool)
        n1134 = xnode "Read/Write Control"("FPGA VI Reference In"=w1718, "error in"=w1717, "Phase count adjustment (Green FB)"=w1715) -> ("FPGA VI Reference Out"=w1713:T19, "error out"=w1714:errorcluster)
        n1135 = xnode "Read/Write Control"("FPGA VI Reference In"=w1713, "error in"=w1714, "+ phase (Green FB)"=w1711) -> ("error out"=w1712:errorcluster)  [unwired: 1 out]
      }
      event "Invert APD Gate", "APD Gate ON Count", "APD Gate OFF Count", "APD Gate", "APD Integration Time (s)", "APD 1 AO Mult.", "APD 2 AO Mult.", "On one out of X cycles": Value Change {
        n1136 = event-data() -> ()  [unwired: 7 out]
        n1137 = Add(x="GI Frequency, ON count", y="GI Frequency, OFF count") -> (x+y=w1722:u32)
        n1138 = Add(x="APD Gate ON Count", y="APD Gate OFF Count") -> (x+y=w1735:u32)
        n1139 = Multiply(x="On one out of X cycles", y=w1722) -> (x*y=w1719:u32)
        "Green FB Count" <- w1719
        n1140 = Subtract(x=w1719, y="GI Frequency, ON count") -> (x-y=w1720:u32)
        n1141 = Multiply(x=w1735, y="On one out of X cycles") -> (x*y=w1734:u32)
        n1142 = Subtract(x=w1734, y="APD Gate ON Count") -> (x-y=w1733:u32)
        n1143 = local read "DMA Update Period (s)"() -> (w1736:dbl)
        n1144 = Multiply(x="APD Integration Time (s)", y=40000000.0) -> (x*y=w1741:dbl)
        n1145 = Reciprocal(x="APD Integration Time (s)") -> (1/x=→"APD Acq Rate (Hz)":dbl)
        n1146 = To Unsigned Long Integer(number=w1741) -> (unsigned 32bit integer=w1725:u32)
        "APD Int. Count" <- w1725
        n1147 = xnode "Read/Write Control"("FPGA VI Reference In"=w1745, "error in"=w1744, "Invert APD Gate"="Invert APD Gate", "APD Gate ON Count"="APD Gate ON Count", "APD Gate OFF Count"=w1733, "APD Acq Rate Count"=w1725, "APD Gate Operating Mode"="APD Gate", "APD 1 AO scale factor"="APD 1 AO Mult.", "APD 2 AO scale factor"="APD 2 AO Mult.", "Green interlace ON count"="GI Frequency, ON count", "Green interlace OFF count"=w1720, "Green interlace ON count 2"="GI Frequency, ON count", "Green interlace OFF count 2"=w1720, "Green FB Count"=w1719) -> ("error out"=w1743:errorcluster)  [unwired: 1 out]
        n1148 = Divide(x=w1736, y="APD Integration Time (s)") -> (x/y=w1739:dbl)
        n1149 = Multiply(x=2.0, y=w1739) -> (x*y=w1738:dbl)
        n1150 = local write "APD Samples/FIFO Acq."(w1739) -> ()
        n1151 = local write "APD Elements/DMA read"(w1738) -> ()
      }
      event "Number of F/B Scans (AOD)", "Scan Speed (nm/s)", "Scan BD", "Initial delta (MHz)", "Step Size (nm)", "Scan Range (nm)": Value Change {
        w1807 = 123.0  # AOM cal (nm/MHz)
        n1152 = event-data() -> ()  [unwired: 7 out]
        n1153 = local read "BD 1 Frequency 1 (MHz)"() -> (w1790:dbl)
        n1154 = local read "AOM X Cal (nm/MHz)"() -> (w1782:dbl)
        n1155 = local read "X RF Frequency Limits (MHz)"() -> (w1794:T16)
        n1156 = local read "Y RF Frequency Limits (MHz)"() -> (w1791:T16)
        n1157 = local read "BD 2 Frequency 1 (MHz)"() -> (w1796:dbl)
        n1158 = Negate(x="Scan Range (nm)") -> (-x=w1760:dbl)
        n1159 = Divide(x=w1760, y=w1782) -> (x/y=w1764:dbl)
        n1160 = Select(t=w1794, s="Scan BD", f=w1791) -> (s? t:f=w1793:T16)
        n1161 = Select(t=w1790, s="Scan BD", f=w1796) -> (s? t:f=w1795:dbl)
        n1162 = Unbundle By Name(w1793) -> ("Maximum"=w1802:dbl, "Minimum"=w1801:dbl)
        n1163 = Add(x=w1764, y=w1795) -> (x+y=w1799:dbl)
        n1164 = Divide(x=w1760, y="Step Size (nm)") -> (x/y=w1779:dbl)
        n1165 = Divide(x="Step Size (nm)", y=w1782) -> (x/y=w1788:dbl)
        n1166 = Absolute Value(x=w1779) -> (abs(x)=w1763:dbl)
        n1167 = Sign(1:w1760) -> (0:w1761:dbl)
        n1168 = In Range and Coerce(upper limit=w1802, x=w1799, lower limit=w1801) -> (coerced(x)=w1798:dbl, In Range?=w1800:bool)
        n1169 = To Unsigned Quad Integer(1:w1763) -> (0:w1778:u64)
        "Scan steps (AOD)" <- w1778
        n1170 = call "IR AOM freq to word.vi"("Frequency In (MHz)"=w1788) -> ("Frequency Word Out (double)"=w1785:dbl)
        n1171 = Multiply(x=w1761, y=w1785) -> (x*y=w1762:dbl)
        n1172 = Subtract(x=w1799, y=w1798) -> (x-y=w1797:dbl)
        n1173 = To Quad Integer(1:w1762) -> (0:w1784:i64)
        "Incr. int (AOD)" <- w1784
        n1174 = Subtract(x=w1764, y=w1797) -> (x-y=w1783:dbl)
        "Scan Range (MHz)" <- w1783
        n1175 = Select(t=w1764, s=w1800, f=w1783) -> (s? t:f=w1803:dbl)
        n1176 = Multiply(x=w1783, y=w1782) -> (x*y=w1781:dbl)
        n1177 = Decrement(x=w1778) -> (x-1=w1831:u64)
        n1178 = Negate(x=w1781) -> (-x=w1777:dbl)
        n1179 = local write "Scan Range (nm)"(w1777) -> ()
        n1180 = Divide(x=w1803, y=w1831) -> (x/y=w1787:dbl)
        "Scan Increment (MHz)" <- w1787
        n1181 = call "IR AOM freq to word.vi"("Frequency In (MHz)"=w1787) -> ("Frequency Word Out (double)"=w1786:dbl)
        n1182 = Divide(x="Step Size (nm)", y="Scan Speed (nm/s)") -> (x/y=w1774:dbl)
        n1183 = To Quad Integer(1:w1786) -> ()  [unwired: 1 out]
        n1184 = local read "Number Interlace Sets"() -> (w1758:u8)
        n1185 = local read "AI Count (ticks)"() -> (w1759:u32)
        n1186 = local read "Total Counts (ticks)"() -> (w1757:u32)
        n1187 = local read "# Samples/trap"() -> (w1789:u32)
        n1188 = Multiply(x=w1759, y=w1758) -> (x*y=w1756:u32)
        n1189 = Divide(x=w1757, y=w1756) -> (x/y=w1755:dbl)
        n1190 = Select(t=w1790, s="Scan BD", f=w1796) -> (s? t:f=w1828:dbl)
        "Initial freq. (MHz)" <- w1828
        n1191 = Add(x=w1803, y=w1828) -> (x+y=→"Final freq. (MHz)":dbl)
        n1192 = Divide(x=w1757, y=40000000.0) -> (x/y=w1773:dbl)
        n1193 = Divide(x=w1774, y=w1773) -> (x/y=w1772:dbl)
        n1194 = To Unsigned Quad Integer(1:w1772) -> (0:w1747:u64)
        n1195 = Quotient & Remainder(x=w1747, y=u64 2) -> (x-y*floor(x/y)=w1751:u64)  [unwired: 1 out]
        n1196 = Equal?(x=w1751, y=u64 0) -> (x = y?=w1749:bool)
        n1197 = Decrement(x=w1747) -> (x-1=w1748:u64)
        n1198 = Select(t=w1747, s=w1749, f=w1748) -> (s? t:f=w1746:u64)
        "Cycles/step (AOD)" <- w1746
        n1199 = xnode "Read/Write Control"("FPGA VI Reference In"=w1839, "error in"=w1838, "Scan steps"=w1778, "Number of scans"="Number of F/B Scans (AOD)", "Cycles per step"=w1746, "Scan freq.  increment"=w1784, "Scan BD"="Scan BD") -> ("error out"=w1837:errorcluster)  [unwired: 1 out]
        n1200 = Multiply(x=w1778, y=w1746) -> (x*y=w1832:u64)
        n1201 = Multiply(x=w1832, y=u64 2) -> (x*y=w1754:u64)
        n1202 = Multiply(x=w1755, y=w1754) -> (x*y=w1753:dbl)
        "Data points/scan (f/b)" <- w1753
        n1203 = Multiply(x=w1753, y="Number of F/B Scans (AOD)") -> (x*y=w1835:dbl)
        "Data points/scans" <- w1835
        n1204 = Divide(x=w1835, y=w1789) -> (x/y=→"N sets should be saved":dbl)
        n1205 = Multiply(x=w1832, y=w1773) -> (x*y=w1771:dbl)
        "Time/Scan (s) (AOD)" <- w1771
        n1206 = Select(t=w1803, s="Scan BD", f=0.0) -> (s? t:f=w1829:dbl)
        n1207 = Select(t=0.0, s="Scan BD", f=w1803) -> (s? t:f=w1825:dbl)
        n1208 = local read "BD 2 Frequency 2 (MHz)"() -> (w1821:dbl)
        n1209 = local read "BD 1 Frequency 2 (MHz)"() -> (w1824:dbl)
        n1210 = Add(x=w1825, y=w1796) -> (x+y=w1822:dbl)
        n1211 = Add(x=w1790, y=w1829) -> (x+y=w1823:dbl)
        n1212 = Multiply(x=w1771, y=2.0) -> (x*y=w1770:dbl)
        n1213 = Multiply(x=w1770, y="Number of F/B Scans (AOD)") -> (x*y=w1767:dbl)
        n1214 = Divide(x=w1767, y=60.0) -> (x/y=→"Time to Finish All (min)":dbl)
        n1215 = Add(x="Trap 2 Bead Size (nm)", y="Trap 1 Bead Size (nm)") -> (x+y=w1811:dbl)
        n1216 = Divide(x=w1811, y=2.0) -> (x/y=w1805:dbl)
        n1217 = local read "Initial delta (MHz)"() -> (w1808:dbl)
        n1218 = Subtract(x=w1822, y=w1821) -> (x-y=w1819:dbl)
        n1219 = Subtract(x=w1823, y=w1824) -> (x-y=w1820:dbl)
        n1220 = Square(x=w1819) -> (x^2=w1818:dbl)
        n1221 = Square(x=w1820) -> (x^2=w1817:dbl)
        n1222 = Add(x=w1817, y=w1818) -> (x+y=w1816:dbl)
        n1223 = Square Root(x=w1816) -> (sqrt(x)=w1815:dbl)
        "Final delta (MHz)" <- w1815
        n1224 = Multiply(x=w1807, y=w1815) -> (x*y=w1814:dbl)
        n1225 = Multiply(x=w1808, y=w1807) -> (x*y=w1806:dbl)
        n1226 = Subtract(x=w1806, y=w1805) -> (x-y=→"Initial sep (nm)":dbl)
        n1227 = Subtract(x=w1814, y=w1805) -> (x-y=→"Final sep (nm)":dbl)
      }
      event "Freq or Amp switch first", "Swap F1 and F2", "Freq switch delay", "Amp switch delay": Value Change {
        n1228 = event-data() -> ()  [unwired: 7 out]
        n1229 = local read "Freq or Amp switch first"() -> (w1840:bool)
        n1230 = local read "Amp switch delay"() -> (w1841:u16)
        n1231 = local read "Freq switch delay"() -> (w1843:u16)
        n1232 = local read "Swap F1 and F2"() -> (w1842:bool)
        n1233 = xnode "Read/Write Control"("FPGA VI Reference In"=w1846, "error in"=w1845, "Freq switch delay"=w1843, "Swap F1 and F2"=w1842, "Amp switch delay"=w1841, "Freq or Amp switch first"=w1840) -> ("error out"=w1844:errorcluster)  [unwired: 1 out]
      }
      event "Scan steps (MCL)", "Number of scans (MCL)", "Scan Range (V)\n(of steps)", "2D or 1D Scan", "N APD Samp/step", "Fast Scan Dir", "Continuous MCL Scanning", "Scan lines (y)": Value Change {
        w1848 = 32767.0 ("y")
        n1234 = event-data() -> ()  [unwired: 7 out]
        n1235 = Select(t="Scan lines (y)", s="2D or 1D Scan", f="Number of scans (MCL)") -> (s? t:f=w1853:u64)
        n1236 = Decrement(x="Scan steps (MCL)") -> (x-1=w1869:u64)
        n1237 = Divide(x="Scan Range (V)\n(of steps)", y=w1869) -> (x/y=w1868:dbl)
        "Desired Scan Incr (V)" <- w1868
        n1238 = local read "APD Integration Time (s)"() -> (w1861:dbl)
        n1239 = Multiply(x=w1868, y=w1848) -> (x*y=w1877:dbl)
        n1240 = Divide(x=w1877, y=10.0) -> (x/y=w1867:dbl)
        "Desired incr (int)" <- w1867
        n1241 = local read "Update Count (MCL)"() -> (w1873:u32)
        n1242 = Round Toward -Infinity(1:w1867) -> (0:w1876:dbl)
        n1243 = To Word Integer(number=w1876) -> (16bit integer=w1851:i16)
        "Actual Incr. int (MCL)" <- w1851
        n1244 = Multiply(x=w1861, y=40000000.0) -> (x*y=w1874:dbl)
        n1245 = Divide(x=w1874, y=w1873) -> (x/y=w1872:dbl)
        n1246 = Multiply(x=i16 10, y=w1851) -> (x*y=w1849:i16)
        n1247 = Multiply(x="N APD Samp/step", y=w1872) -> (x*y=w1871:dbl)
        "Cycles/step (MCL)" <- w1871
        n1248 = Divide(x=w1849, y=w1848) -> (x/y=→"Actual MCL Inc (V)":dbl)
        n1249 = Multiply(x="N APD Samp/step", y="Scan steps (MCL)") -> (x*y=w1863:dbl)
        n1250 = local read "APD Samples/FIFO Acq."() -> (w1860:dbl)
        n1251 = Multiply(x=w1863, y=u64 2) -> (x*y=w1862:dbl)
        "Data points/scan (f+b)" <- w1862
        n1252 = Multiply(x=w1862, y=w1853) -> (x*y=w1880:dbl)
        "Data points/scans (MCL)" <- w1880
        n1253 = Multiply(x=w1861, y=w1862) -> (x*y=w1854:dbl)
        "Time/f+b scan (s) (MCL)" <- w1854
        n1254 = Divide(x=w1880, y=w1860) -> (x/y=→"N sets should be saved (MCL)":dbl)
        n1255 = Multiply(x=w1854, y=w1853) -> (x*y=→"Total Time (s)":dbl)
        n1256 = Not(x="Fast Scan Dir") -> (.not. x?=w1858:bool)
        n1257 = xnode "Read/Write Control"("FPGA VI Reference In"=w1884, "error in"=w1883, "Scan steps (MCL)"="Scan steps (MCL)", "Number of scans (MCL)"=w1853, "Cycles per step (MCL)"=w1871, "Scan freq.  increment (MCL)"=w1851, "1D or 2D Scan?"="2D or 1D Scan", "MCL Scan Axis"=w1858, "Cont. Scan (MCL)"="Continuous MCL Scanning") -> ("error out"=w1882:errorcluster)  [unwired: 1 out]
      }
      event "Read Cal": Value Change {
        w1886 = 1000.0 ("y")
        n1258 = event-data() -> ()  [unwired: 7 out]
        n1259 = local read "Save file name"() -> (w1911:path)
        n1260 = local write "Read Cal"(FALSE ("Read Cal")) -> ()
        n1261 = Strip Path(path=w1911) -> (stripped path=w1910:path)  [unwired: 1 out]
        n1262 = Path To String(path=w1910) -> (string=w1909:string)
        n1263 = Concatenate Strings(w1909, "\\current.cal" ("string")) -> (w1907:string)
        n1264 = String To Path(string=w1907) -> (path=w1906:path)
